vi "Apply Selected Labels to Control.vi"(8 "error in (no error)":errorcluster, 10 "Alternate Text Select (0)":i32, 11 "Tab in":refnum<class "Tab.lvclass">) -> (0 "error out":errorcluster, 3 "Tab out":refnum<class "Tab.lvclass">)   [LabVIEW 2017, in "Localization.lvlib" / "Tab.lvclass"]
doc: "Use the information in the class to apply the selected alternate text from the Additional Labels to the control.\n\nChoose Movement Consulting, LLC"
uses:
  Tab.lvclass
  C:/Apps/CMC/OpenSource/Localization/Control Info/Control Info.lvclass
  Control Info/Control Info.lvclass
  Localization.lvlib
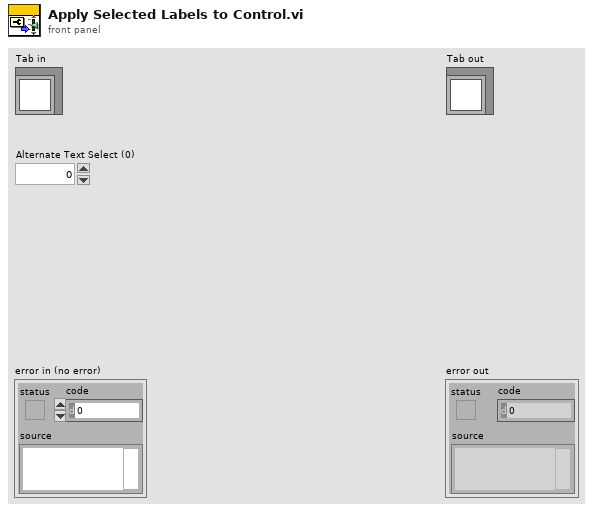
[diagram p1: front panel]
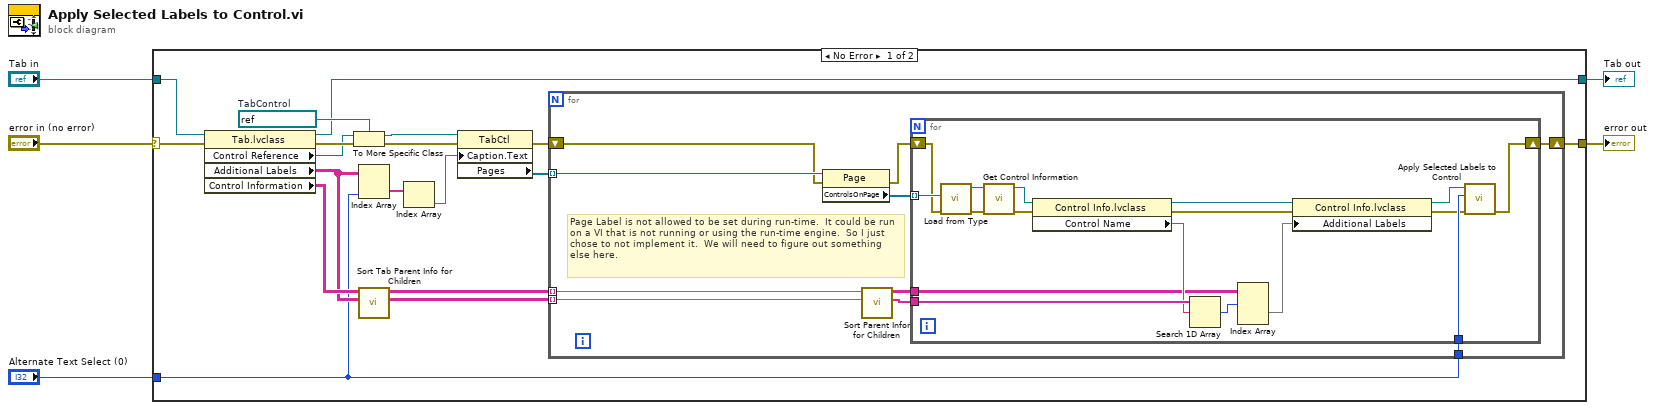
[diagram p0: block diagram]
diagram:
  n1 = case shown="No Error" "error in (no error)" {
    selector: "error in (no error)" -> [w18 w52]
    tunnel: "Tab in" -> [w17 w51]
    tunnel: [w7 w52] -> w1
    tunnel: [w14 w51] -> w2
    tunnel: "Alternate Text Select (0)" -> [w6 _]
    frame No Error {
      w23 = refnum<vi> refnum  # TabControl
      n2 = property class="Tab.lvclass"(reference=w17, error in=w18) -> (reference out=w14:refnum<class "Tab.lvclass">, error out=w20:errorcluster, "Control Reference"=w19:refnum<vi>, "Additional Labels"=w11:string[][], "Control Information"=w12:string[][])
      n3 = To More Specific Class(target class=w23, reference=w19, error in=w20) -> (specific class reference=w22:refnum<vi>, error out=w21:errorcluster)
      n4 = Index Array(array=w11, index (col)=w6) -> (element=w15:string[])  [unwired: 1 in]
      n5 = call "Sort Tab Parent Info for Children.vi"("Additional Labels"=w11, "Control Information in"=w12) -> ("Broken Out Additional Labels"=w10:string[][][], "Control Info by Page"=w9:string[][][])  [unwired: 7 in, 1 out]
      n6 = Index Array(array=w15) -> (element=w16:string)  [unwired: 1 in]
      n7 = property class="TabCtl"(reference=w22, error in=w21, "Caption.Text"=w16) -> (error out=w8:errorcluster, "Pages"=w13:refnum<vi>[])  [unwired: 1 out]
      n8 = for {
        tunnel: w13 -> [w31] mode=indexing
        tunnel: w6 -> [w33]
        tunnel: w10 -> [w24] mode=indexing
        tunnel: w9 -> [w27] mode=indexing
        shift-right: [w32] -> w7
        shift-left: w8 -> [w29]
        # "Page Label is not allowed to be set during run-time.  It could be run on a VI that is not running or using the run-time engine.  So I just chose to not implement it.  We will need to figure out something else here."
        n9 = property class="Page"(reference=w31, error in=w29) -> (error out=w28:errorcluster, "ControlsOnPage"=w30:refnum<vi>[])  [unwired: 1 out]
        n10 = call "Sort Parent Infor for Children.vi"("Additional Labels"=w24, "Control Information in"=w27) -> ("Control Names"=w25:string[], "Broken Out Additional Labels"=w26:string[][][])  [unwired: 7 in, 1 out]
        n11 = for {
          tunnel: w30 -> [w50] mode=indexing
          tunnel: w33 -> [w49]
          tunnel: w25 -> [w46]
          tunnel: w26 -> [w44]
          shift-right: [w39] -> w32
          shift-left: w28 -> [w34]
          n12 = call "Load from Type.vi"("error in (no error)"=w34, "Control Reference"=w50) -> ("error out"=w37:errorcluster, "Control Info out"=w38:refnum<class "Control Info.lvclass">)  [unwired: 8 in]
          n13 = call-dynamic "Get Control Information.vi"("error in (no error)"=w37, "Control Info in"=w38) -> ("error out"=w36:errorcluster, "Control Info out"=w35:refnum<class "Control Info.lvclass">)  [unwired: 7 in, 1 out]
          n14 = property class="Control Info.lvclass"(reference=w35, error in=w36) -> (reference out=w47:refnum<class "Control Info.lvclass">, error out=w48:errorcluster, "Control Name"=w45:string)
          n15 = Search 1D Array(1D array=w46, element=w45) -> (index of element=w43:i32)  [unwired: 1 in]
          n16 = Index Array(array=w44, index (dim 0)=w43) -> (element=w42:string[][])  [unwired: 2 in]
          n17 = property class="Control Info.lvclass"(reference=w47, error in=w48, "Additional Labels"=w42) -> (reference out=w40:refnum<class "Control Info.lvclass">, error out=w41:errorcluster)
          n18 = call-dynamic "Apply Selected Labels to Control.vi"("error in (no error)"=w41, "Alternate Text Select (0)"=w49, "Control Info in"=w40) -> ("error out"=w39:errorcluster)  [unwired: 7 in, 1 out]
        }
      }
    }
    frame Error {
    }
  }
  "error out" <- w1
  "Tab out" <- w2
